vi "Really Big Cluster.vi"(1 "Cluster":T1) -> (0 "Cluster out":T1)   [LabVIEW 2012]
types:
  T1 = cluster{"Numeric":u32, "Numeric 2":u32, "Numeric 3":u32, "Numeric 4":u32, "Numeric 5":u32, "Numeric 6":u32, "Numeric 7":u32, "Numeric 8":u32, "Numeric 9":u32, "Numeric 10":u32, "Numeric 11":u32, "Numeric 12":u32, "Numeric 13":u32, "Numeric 14":u32, "Numeric 15":u32, "Numeric 16":u32, "Numeric 17":u32, "Numeric 18":u32, "Numeric 19":u32, "Numeric 20":u32, "Numeric 21":u32, "Numeric 22":u32, "Numeric 23":u32, "Numeric 24":u32, "Numeric 25":u32, "Numeric 26":u32, "Numeric 27":u32, "Numeric 28":u32, "Numeric 29":u32, "Numeric 30":u32, "Numeric 31":u32, "Numeric 32":u32, "Numeric 33":u32, "Numeric 34":u32, "Numeric 35":u32, "Numeric 36":u32, "Numeric 37":u32, "Numeric 38":u32, "Numeric 39":u32, "Numeric 40":u32, "Numeric 41":u32, "Numeric 42":u32, "Numeric 43":u32, "Numeric 44":u32, "Numeric 45":u32, "Numeric 46":u32, "Numeric 47":u32, "Numeric 48":u32, "Numeric 49":u32, "Numeric 50":u32, "Numeric 51":u32, "Numeric 52":u32, "Numeric 53":u32, "Numeric 54":u32, "Numeric 55":u32, "Numeric 56":u32, "Numeric 57":u32, "Numeric 58":u32, "Numeric 59":u32, "Numeric 60":u32, "Numeric 61":u32, "Numeric 62":u32, "Numeric 63":u32, "Numeric 64":u32, "Numeric 65":u32, "Numeric 66":u32, "Numeric 67":u32, "Numeric 68":u32, "Numeric 69":u32, "Numeric 70":u32, "Numeric 71":u32, "Numeric 72":u32, "Numeric 73":u32, "Numeric 74":u32, "Numeric 75":u32, "Numeric 76":u32, "Numeric 77":u32, "Numeric 78":u32, "Numeric 79":u32, "Numeric 80":u32, "Numeric 81":u32, "Numeric 82":u32, "Numeric 83":u32, "Numeric 84":u32, "Numeric 85":u32, "Numeric 86":u32, "Numeric 87":u32, "Numeric 88":u32, "Numeric 89":u32, "Numeric 90":u32, "Numeric 91":u32, "Numeric 92":u32, "Numeric 93":u32, "Numeric 94":u32, "Numeric 95":u32, "Numeric 96":u32, "Numeric 97":u32, "Numeric 98":u32, "Numeric 99":u32, "Numeric 100":u32, "Numeric 101":u32, "Numeric 102":u32, "Numeric 103":u32, "Numeric 104":u32, "Numeric 105":u32, "Numeric 106":u32, "Numeric 107":u32, "Numeric 108":u32, "Numeric 109":u32, "Numeric 110":u32, "Numeric 111":u32, "Numeric 112":u32, "Numeric 113":u32, "Numeric 114":u32, "Numeric 115":u32, "Numeric 116":u32, "Numeric 117":u32, "Numeric 118":u32, "Numeric 119":u32, "Numeric 120":u32, "Numeric 121":u32, "Numeric 122":u32, "Numeric 123":u32, "Numeric 124":u32, "Numeric 125":u32, "Numeric 126":u32, "Numeric 127":u32, "Numeric 128":u32, "Numeric 129":u32, "Numeric 130":u32, "Numeric 131":u32, "Numeric 132":u32, "Numeric 133":u32, "Numeric 134":u32, "Numeric 135":u32, "Numeric 136":u32, "Numeric 137":u32, "Numeric 138":u32, "Numeric 139":u32, "Numeric 140":u32, "Numeric 141":u32, "Numeric 142":u32, "Numeric 143":u32, "Numeric 144":u32, "Numeric 145":u32, "Numeric 146":u32, "Numeric 147":u32, "Numeric 148":u32, "Numeric 149":u32, "Numeric 150":u32, "Numeric 151":u32, "Numeric 152":u32, "Numeric 153":u32, "Numeric 154":u32, "Numeric 155":u32, "Numeric 156":u32, "Numeric 157":u32, "Numeric 158":u32, "Numeric 159":u32, "Numeric 160":u32, "Numeric 161":u32, "Numeric 162":u32, "Numeric 163":u32, "Numeric 164":u32, "Numeric 165":u32, "Numeric 166":u32, "Numeric 167":u32, "Numeric 168":u32, "Numeric 169":u32, "Numeric 170":u32, "Numeric 171":u32, "Numeric 172":u32, "Numeric 173":u32, "Numeric 174":u32, "Numeric 175":u32, "Numeric 176":u32, "Numeric 177":u32, "Numeric 178":u32, "Numeric 179":u32, "Numeric 180":u32, "Numeric 181":u32, "Numeric 182":u32, "Numeric 183":u32, "Numeric 184":u32, "Numeric 185":u32, "Numeric 186":u32, "Numeric 187":u32, "Numeric 188":u32, "Numeric 189":u32, "Numeric 190":u32, "Numeric 191":u32, "Numeric 192":u32, "Numeric 193":u32, "Numeric 194":u32, "Numeric 195":u32, "Numeric 196":u32, "Numeric 197":u32, "Numeric 198":u32, "Numeric 199":u32, "Numeric 200":u32, "Numeric 201":u32, "Numeric 202":u32, "Numeric 203":u32, "Numeric 204":u32, "Numeric 205":u32, "Numeric 206":u32, "Numeric 207":u32, "Numeric 208":u32, "Numeric 209":u32, "Numeric 210":u32, "Numeric 211":u32, "Numeric 212":u32, "Numeric 213":u32, "Numeric 214":u32, "Numeric 215":u32, "Numeric 216":u32, "Numeric 217":u32, "Numeric 218":u32, "Numeric 219":u32, "Numeric 220":u32, "Numeric 221":u32, "Numeric 222":u32, "Numeric 223":u32, "Numeric 224":u32, "Numeric 225":u32, "Numeric 226":u32, "Numeric 227":u32, "Numeric 228":u32, "Numeric 229":u32, "Numeric 230":u32, "Numeric 231":u32, "Numeric 232":u32, "Numeric 233":u32, "Numeric 234":u32, "Numeric 235":u32, "Numeric 236":u32, "Numeric 237":u32, "Numeric 238":u32, "Numeric 239":u32, "Numeric 240":u32, "Numeric 241":u32, "Numeric 242":u32, "Numeric 243":u32, "Numeric 244":u32, "Numeric 245":u32, "Numeric 246":u32, "Numeric 247":u32, "Numeric 248":u32, "Numeric 249":u32, "Numeric 250":u32, "Numeric 251":u32, "Numeric 252":u32, "Numeric 253":u32, "Numeric 254":u32, "Numeric 255":u32, "Numeric 256":u32, "Numeric 257":u32, "Numeric 258":u32, "Numeric 259":u32, "Numeric 260":u32, "Numeric 261":u32, "Numeric 262":u32, "Numeric 263":u32, "Numeric 264":u32, "Numeric 265":u32, "Numeric 266":u32, "Numeric 267":u32, "Numeric 268":u32, "Numeric 269":u32, "Numeric 270":u32, "Numeric 271":u32, "Numeric 272":u32, "Numeric 273":u32, "Numeric 274":u32, "Numeric 275":u32, "Numeric 276":u32, "Numeric 277":u32, "Numeric 278":u32, "Numeric 279":u32, "Numeric 280":u32, "Numeric 281":u32, "Numeric 282":u32, "Numeric 283":u32, "Numeric 284":u32, "Numeric 285":u32, "Numeric 286":u32, "Numeric 287":u32, "Numeric 288":u32, "Numeric 289":u32, "Numeric 290":u32, "Numeric 291":u32, "Numeric 292":u32, "Numeric 293":u32, "Numeric 294":u32, "Numeric 295":u32, "Numeric 296":u32, "Numeric 297":u32, "Numeric 298":u32, "Numeric 299":u32, "Numeric 300":u32, "Numeric 301":u32, "Numeric 302":u32, "Numeric 303":u32, "Numeric 304":u32, "Numeric 305":u32, "Numeric 306":u32, "Numeric 307":u32, "Numeric 308":u32, "Numeric 309":u32, "Numeric 310":u32, "Numeric 311":u32, "Numeric 312":u32, "Numeric 313":u32, "Numeric 314":u32, "Numeric 315":u32, "Numeric 316":u32, "Numeric 317":u32, "Numeric 318":u32, "Numeric 319":u32, "Numeric 320":u32, "Numeric 321":u32, "Numeric 322":u32, "Numeric 323":u32, "Numeric 324":u32, "Numeric 325":u32, "Numeric 326":u32, "Numeric 327":u32, "Numeric 328":u32, "Numeric 329":u32, "Numeric 330":u32, "Numeric 331":u32, "Numeric 332":u32, "Numeric 333":u32, "Numeric 334":u32, "Numeric 335":u32, "Numeric 336":u32, "Numeric 337":u32, "Numeric 338":u32, "Numeric 339":u32, "Numeric 340":u32, "Numeric 341":u32, "Numeric 342":u32, "Numeric 343":u32, "Numeric 344":u32, "Numeric 345":u32, "Numeric 346":u32, "Numeric 347":u32, "Numeric 348":u32, "Numeric 349":u32, "Numeric 350":u32, "Numeric 351":u32, "Numeric 352":u32, "Numeric 353":u32, "Numeric 354":u32, "Numeric 355":u32, "Numeric 356":u32, "Numeric 357":u32, "Numeric 358":u32, "Numeric 359":u32, "Numeric 360":u32, "Numeric 361":u32, "Numeric 362":u32, "Numeric 363":u32, "Numeric 364":u32, "Numeric 365":u32, "Numeric 366":u32, "Numeric 367":u32, "Numeric 368":u32, "Numeric 369":u32, "Numeric 370":u32, "Numeric 371":u32, "Numeric 372":u32, "Numeric 373":u32, "Numeric 374":u32, "Numeric 375":u32, "Numeric 376":u32, "Numeric 377":u32, "Numeric 378":u32, "Numeric 379":u32, "Numeric 380":u32, "Numeric 381":u32, "Numeric 382":u32, "Numeric 383":u32, "Numeric 384":u32, "Numeric 385":u32, "Numeric 386":u32, "Numeric 387":u32, "Numeric 388":u32, "Numeric 389":u32, "Numeric 390":u32, "Numeric 391":u32, "Numeric 392":u32, "Numeric 393":u32, "Numeric 394":u32, "Numeric 395":u32, "Numeric 396":u32, "Numeric 397":u32, "Numeric 398":u32, "Numeric 399":u32, "Numeric 400":u32, "Numeric 401":u32, "Numeric 402":u32, "Numeric 403":u32, "Numeric 404":u32, "Numeric 405":u32, "Numeric 406":u32, "Numeric 407":u32, "Numeric 408":u32, "Numeric 409":u32, "Numeric 410":u32, "Numeric 411":u32, "Numeric 412":u32, "Numeric 413":u32, "Numeric 414":u32, "Numeric 415":u32, "Numeric 416":u32, "Numeric 417":u32, "Numeric 418":u32, "Numeric 419":u32, "Numeric 420":u32, "Numeric 421":u32, "Numeric 422":u32, "Numeric 423":u32, "Numeric 424":u32, "Numeric 425":u32, "Numeric 426":u32, "Numeric 427":u32, "Numeric 428":u32, "Numeric 429":u32, "Numeric 430":u32, "Numeric 431":u32, "Numeric 432":u32, "Numeric 433":u32, "Numeric 434":u32, "Numeric 435":u32, "Numeric 436":u32, "Numeric 437":u32, "Numeric 438":u32, "Numeric 439":u32, "Numeric 440":u32, "Numeric 441":u32, "Numeric 442":u32, "Numeric 443":u32, "Numeric 444":u32, "Numeric 445":u32, "Numeric 446":u32, "Numeric 447":u32, "Numeric 448":u32, "Numeric 449":u32, "Numeric 450":u32, "Numeric 451":u32, "Numeric 452":u32, "Numeric 453":u32, "Numeric 454":u32, "Numeric 455":u32, "Numeric 456":u32, "Numeric 457":u32, "Numeric 458":u32, "Numeric 459":u32, "Numeric 460":u32, "Numeric 461":u32, "Numeric 462":u32, "Numeric 463":u32, "Numeric 464":u32, "Numeric 465":u32, "Numeric 466":u32, "Numeric 467":u32, "Numeric 468":u32, "Numeric 469":u32, "Numeric 470":u32, "Numeric 471":u32, "Numeric 472":u32, "Numeric 473":u32, "Numeric 474":u32, "Numeric 475":u32, "Numeric 476":u32, "Numeric 477":u32, "Numeric 478":u32, "Numeric 479":u32, "Numeric 480":u32, "Numeric 481":u32, "Numeric 482":u32, "Numeric 483":u32, "Numeric 484":u32, "Numeric 485":u32, "Numeric 486":u32, "Numeric 487":u32, "Numeric 488":u32, "Numeric 489":u32, "Numeric 490":u32, "Numeric 491":u32, "Numeric 492":u32, "Numeric 493":u32, "Numeric 494":u32, "Numeric 495":u32, "Numeric 496":u32, "Numeric 497":u32, "Numeric 498":u32, "Numeric 499":u32, "Numeric 500":u32, "Numeric 501":u32, "Numeric 502":u32, "Numeric 503":u32, "Numeric 504":u32, "Numeric 505":u32, "Numeric 506":u32, "Numeric 507":u32, "Numeric 508":u32, "Numeric 509":u32, "Numeric 510":u32, "Numeric 511":u32, "Numeric 512":u32, "Numeric 513":u32, "Numeric 514":u32, "Numeric 515":u32, "Numeric 516":u32, "Numeric 517":u32, "Numeric 518":u32, "Numeric 519":u32, "Numeric 520":u32, "Numeric 521":u32, "Numeric 522":u32, "Numeric 523":u32, "Numeric 524":u32, "Numeric 525":u32, "Numeric 526":u32, "Numeric 527":u32, "Numeric 528":u32, "Numeric 529":u32, "Numeric 530":u32, "Numeric 531":u32, "Numeric 532":u32, "Numeric 533":u32, "Numeric 534":u32, "Numeric 535":u32, "Numeric 536":u32, "Numeric 537":u32, "Numeric 538":u32, "Numeric 539":u32, "Numeric 540":u32, "Numeric 541":u32, "Numeric 542":u32, "Numeric 543":u32, "Numeric 544":u32, "Numeric 545":u32, "Numeric 546":u32, "Numeric 547":u32, "Numeric 548":u32, "Numeric 549":u32, "Numeric 550":u32, "Numeric 551":u32, "Numeric 552":u32, "Numeric 553":u32, "Numeric 554":u32, "Numeric 555":u32, "Numeric 556":u32, "Numeric 557":u32, "Numeric 558":u32, "Numeric 559":u32, "Numeric 560":u32, "Numeric 561":u32, "Numeric 562":u32, "Numeric 563":u32, "Numeric 564":u32, "Numeric 565":u32, "Numeric 566":u32, "Numeric 567":u32, "Numeric 568":u32, "Numeric 569":u32, "Numeric 570":u32, "Numeric 571":u32, "Numeric 572":u32, "Numeric 573":u32, "Numeric 574":u32, "Numeric 575":u32, "Numeric 576":u32, "Numeric 577":u32, "Numeric 578":u32, "Numeric 579":u32, "Numeric 580":u32, "Numeric 581":u32, "Numeric 582":u32, "Numeric 583":u32, "Numeric 584":u32, "Numeric 585":u32, "Numeric 586":u32, "Numeric 587":u32, "Numeric 588":u32, "Numeric 589":u32, "Numeric 590":u32, "Numeric 591":u32, "Numeric 592":u32, "Numeric 593":u32, "Numeric 594":u32, "Numeric 595":u32, "Numeric 596":u32, "Numeric 597":u32, "Numeric 598":u32, "Numeric 599":u32, "Numeric 600":u32, "Numeric 601":u32, "Numeric 602":u32, "Numeric 603":u32, "Numeric 604":u32, "Numeric 605":u32, "Numeric 606":u32, "Numeric 607":u32, "Numeric 608":u32, "Numeric 609":u32, "Numeric 610":u32, "Numeric 611":u32, "Numeric 612":u32, "Numeric 613":u32, "Numeric 614":u32, "Numeric 615":u32, "Numeric 616":u32, "Numeric 617":u32, "Numeric 618":u32, "Numeric 619":u32, "Numeric 620":u32, "Numeric 621":u32, "Numeric 622":u32, "Numeric 623":u32, "Numeric 624":u32, "Numeric 625":u32, "Numeric 626":u32, "Numeric 627":u32, "Numeric 628":u32, "Numeric 629":u32, "Numeric 630":u32, "Numeric 631":u32, "Numeric 632":u32, "Numeric 633":u32, "Numeric 634":u32, "Numeric 635":u32, "Numeric 636":u32, "Numeric 637":u32, "Numeric 638":u32, "Numeric 639":u32, "Numeric 640":u32, "Numeric 641":u32, "Numeric 642":u32, "Numeric 643":u32, "Numeric 644":u32, "Numeric 645":u32, "Numeric 646":u32, "Numeric 647":u32, "Numeric 648":u32, "Numeric 649":u32, "Numeric 650":u32, "Numeric 651":u32, "Numeric 652":u32, "Numeric 653":u32, "Numeric 654":u32, "Numeric 655":u32, "Numeric 656":u32, "Numeric 657":u32, "Numeric 658":u32, "Numeric 659":u32, "Numeric 660":u32, "Numeric 661":u32, "Numeric 662":u32, "Numeric 663":u32, "Numeric 664":u32, "Numeric 665":u32, "Numeric 666":u32, "Numeric 667":u32, "Numeric 668":u32, "Numeric 669":u32, "Numeric 670":u32, "Numeric 671":u32, "Numeric 672":u32, "Numeric 673":u32, "Numeric 674":u32, "Numeric 675":u32, "Numeric 676":u32, "Numeric 677":u32, "Numeric 678":u32, "Numeric 679":u32, "Numeric 680":u32, "Numeric 681":u32, "Numeric 682":u32, "Numeric 683":u32, "Numeric 684":u32, "Numeric 685":u32, "Numeric 686":u32, "Numeric 687":u32, "Numeric 688":u32, "Numeric 689":u32, "Numeric 690":u32, "Numeric 691":u32, "Numeric 692":u32, "Numeric 693":u32, "Numeric 694":u32, "Numeric 695":u32, "Numeric 696":u32, "Numeric 697":u32, "Numeric 698":u32, "Numeric 699":u32, "Numeric 700":u32, "Numeric 701":u32, "Numeric 702":u32, "Numeric 703":u32, "Numeric 704":u32, "Numeric 705":u32, "Numeric 706":u32, "Numeric 707":u32, "Numeric 708":u32, "Numeric 709":u32, "Numeric 710":u32, "Numeric 711":u32, "Numeric 712":u32, "Numeric 713":u32, "Numeric 714":u32, "Numeric 715":u32, "Numeric 716":u32, "Numeric 717":u32, "Numeric 718":u32, "Numeric 719":u32, "Numeric 720":u32, "Numeric 721":u32, "Numeric 722":u32, "Numeric 723":u32, "Numeric 724":u32, "Numeric 725":u32, "Numeric 726":u32, "Numeric 727":u32, "Numeric 728":u32, "Numeric 729":u32, "Numeric 730":u32, "Numeric 731":u32, "Numeric 732":u32, "Numeric 733":u32, "Numeric 734":u32, "Numeric 735":u32, "Numeric 736":u32, "Numeric 737":u32, "Numeric 738":u32, "Numeric 739":u32, "Numeric 740":u32, "Numeric 741":u32, "Numeric 742":u32, "Numeric 743":u32, "Numeric 744":u32, "Numeric 745":u32, "Numeric 746":u32, "Numeric 747":u32, "Numeric 748":u32, "Numeric 749":u32, "Numeric 750":u32, "Numeric 751":u32, "Numeric 752":u32, "Numeric 753":u32, "Numeric 754":u32, "Numeric 755":u32, "Numeric 756":u32, "Numeric 757":u32, "Numeric 758":u32, "Numeric 759":u32, "Numeric 760":u32, "Numeric 761":u32, "Numeric 762":u32, "Numeric 763":u32, "Numeric 764":u32, "Numeric 765":u32, "Numeric 766":u32, "Numeric 767":u32, "Numeric 768":u32, "Numeric 769":u32, "Numeric 770":u32, "Numeric 771":u32, "Numeric 772":u32, "Numeric 773":u32, "Numeric 774":u32, "Numeric 775":u32, "Numeric 776":u32, "Numeric 777":u32, "Numeric 778":u32, "Numeric 779":u32, "Numeric 780":u32, "Numeric 781":u32, "Numeric 782":u32, "Numeric 783":u32, "Numeric 784":u32, "Numeric 785":u32, "Numeric 786":u32, "Numeric 787":u32, "Numeric 788":u32, "Numeric 789":u32, "Numeric 790":u32, "Numeric 791":u32, "Numeric 792":u32, "Numeric 793":u32, "Numeric 794":u32, "Numeric 795":u32, "Numeric 796":u32, "Numeric 797":u32, "Numeric 798":u32, "Numeric 799":u32, "Numeric 800":u32, "Numeric 801":u32, "Numeric 802":u32, "Numeric 803":u32, "Numeric 804":u32, "Numeric 805":u32, "Numeric 806":u32, "Numeric 807":u32, "Numeric 808":u32, "Numeric 809":u32, "Numeric 810":u32, "Numeric 811":u32, "Numeric 812":u32, "Numeric 813":u32, "Numeric 814":u32, "Numeric 815":u32, "Numeric 816":u32, "Numeric 817":u32, "Numeric 818":u32, "Numeric 819":u32, "Numeric 820":u32, "Numeric 821":u32, "Numeric 822":u32, "Numeric 823":u32, "Numeric 824":u32, "Numeric 825":u32, "Numeric 826":u32, "Numeric 827":u32, "Numeric 828":u32, "Numeric 829":u32, "Numeric 830":u32, "Numeric 831":u32, "Numeric 832":u32, "Numeric 833":u32, "Numeric 834":u32, "Numeric 835":u32, "Numeric 836":u32, "Numeric 837":u32, "Numeric 838":u32, "Numeric 839":u32, "Numeric 840":u32, "Numeric 841":u32, "Numeric 842":u32, "Numeric 843":u32, "Numeric 844":u32, "Numeric 845":u32, "Numeric 846":u32, "Numeric 847":u32, "Numeric 848":u32, "Numeric 849":u32, "Numeric 850":u32, "Numeric 851":u32, "Numeric 852":u32, "Numeric 853":u32, "Numeric 854":u32, "Numeric 855":u32, "Numeric 856":u32, "Numeric 857":u32, "Numeric 858":u32, "Numeric 859":u32, "Numeric 860":u32, "Numeric 861":u32, "Numeric 862":u32, "Numeric 863":u32, "Numeric 864":u32, "Numeric 865":u32, "Numeric 866":u32, "Numeric 867":u32, "Numeric 868":u32, "Numeric 869":u32, "Numeric 870":u32, "Numeric 871":u32, "Numeric 872":u32, "Numeric 873":u32, "Numeric 874":u32, "Numeric 875":u32, "Numeric 876":u32, "Numeric 877":u32, "Numeric 878":u32, "Numeric 879":u32, "Numeric 880":u32, "Numeric 881":u32, "Numeric 882":u32, "Numeric 883":u32, "Numeric 884":u32, "Numeric 885":u32, "Numeric 886":u32, "Numeric 887":u32, "Numeric 888":u32, "Numeric 889":u32, "Numeric 890":u32, "Numeric 891":u32, "Numeric 892":u32, "Numeric 893":u32, "Numeric 894":u32, "Numeric 895":u32, "Numeric 896":u32, "Numeric 897":u32, "Numeric 898":u32, "Numeric 899":u32, "Numeric 900":u32, "Numeric 901":u32, "Numeric 902":u32, "Numeric 903":u32, "Numeric 904":u32, "Numeric 905":u32, "Numeric 906":u32, "Numeric 907":u32, "Numeric 908":u32, "Numeric 909":u32, "Numeric 910":u32, "Numeric 911":u32, "Numeric 912":u32, "Numeric 913":u32, "Numeric 914":u32, "Numeric 915":u32, "Numeric 916":u32, "Numeric 917":u32, "Numeric 918":u32, "Numeric 919":u32, "Numeric 920":u32, "Numeric 921":u32, "Numeric 922":u32, "Numeric 923":u32, "Numeric 924":u32, "Numeric 925":u32, "Numeric 926":u32, "Numeric 927":u32, "Numeric 928":u32, "Numeric 929":u32, "Numeric 930":u32, "Numeric 931":u32, "Numeric 932":u32, "Numeric 933":u32, "Numeric 934":u32, "Numeric 935":u32, "Numeric 936":u32, "Numeric 937":u32, "Numeric 938":u32, "Numeric 939":u32, "Numeric 940":u32, "Numeric 941":u32, "Numeric 942":u32, "Numeric 943":u32, "Numeric 944":u32, "Numeric 945":u32, "Numeric 946":u32, "Numeric 947":u32, "Numeric 948":u32, "Numeric 949":u32, "Numeric 950":u32, "Numeric 951":u32, "Numeric 952":u32, "Numeric 953":u32, "Numeric 954":u32, "Numeric 955":u32, "Numeric 956":u32, "Numeric 957":u32, "Numeric 958":u32, "Numeric 959":u32, "Numeric 960":u32, "Numeric 961":u32, "Numeric 962":u32, "Numeric 963":u32, "Numeric 964":u32, "Numeric 965":u32, "Numeric 966":u32, "Numeric 967":u32, "Numeric 968":u32, "Numeric 969":u32, "Numeric 970":u32, "Numeric 971":u32, "Numeric 972":u32, "Numeric 973":u32, "Numeric 974":u32, "Numeric 975":u32, "Numeric 976":u32, "Numeric 977":u32, "Numeric 978":u32, "Numeric 979":u32, "Numeric 980":u32, "Numeric 981":u32, "Numeric 982":u32, "Numeric 983":u32, "Numeric 984":u32, "Numeric 985":u32, "Numeric 986":u32, "Numeric 987":u32, "Numeric 988":u32, "Numeric 989":u32, "Numeric 990":u32, "Numeric 991":u32, "Numeric 992":u32, "Numeric 993":u32, "Numeric 994":u32, "Numeric 995":u32, "Numeric 996":u32, "Numeric 997":u32, "Numeric 998":u32, "Numeric 999":u32, "Numeric 1000":u32}
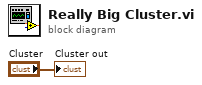
[diagram p0: block diagram]
diagram:
  "Cluster out" <- "Cluster"
